vi "PDE_Cal 3D Pic Color.vi"(11 "U(x, y)":dbl[](array[numeric])) -> (3 "Color Array":T1[](array[typedef]))   [LabVIEW 2020, in "NI_PDE.lvlib"]
uses:
  <vilib>/gmath/NI_PDE.lvlib
  <vilib>/Utility/miscctls.llb/LVRGBAColorTypeDef.ctl
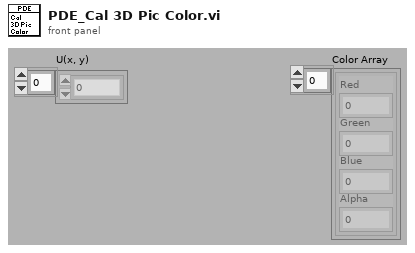
[diagram p1: front panel]
types:
  T1 = typedef "LVRGBAColorTypeDef.ctl" = cluster{"Red":sgl, "Green":sgl, "Blue":sgl, "Alpha":sgl}
  T2 = cluster{"[0]":dbl, "[1]":dbl, "[2]":dbl, "[3]":dbl}
  T3 = cluster{"[0]":dbl, "[1]":dbl, "[2]":dbl, "[3]":dbl}[]
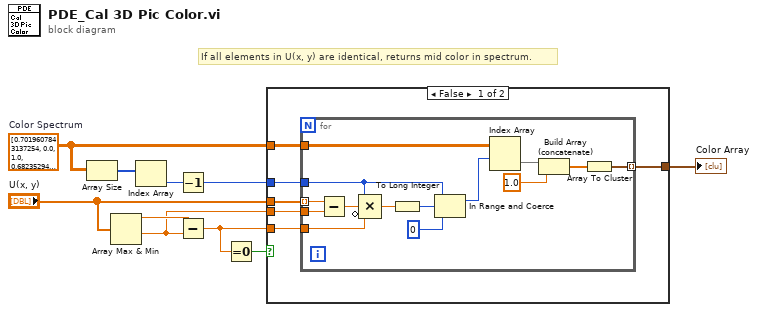
[diagram p0: block diagram]
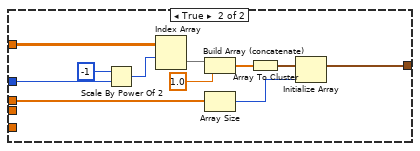
[diagram p2: hidden frame]
diagram:
  w1 = dbl[][] [[0.7019607843137254, 0.0, 1.0], [0.6823529411764706, 0.0, 1.0], [0.6666666666666666, 0.0, 1.0], [0.6470588235294118, 0.0, 1.0], [0.6313725490196078, 0.0, 1.0], [0.611764705882353, 0.0, 1.0], [0.596078431372549, 0.0, 1.0], [0.5803921568627451, 0.0, 1.0], [0.5607843137254902, 0.0, 1.0], [0.5450980392156862, 0.0, 1.0], [0.5254901960784314, 0.0, 1.0], [0.5098039215686274, 0.0, 1.0], [0.49411764705882355, 0.0, 1.0], [0.4745098039215686, 0.0, 1.0], [0.4588235294117647, 0.0, 1.0], [0.44313725490196076, 0.0, 1.0], [0.4235294117647059, 0.0, 1.0], [0.40784313725490196, 0.0, 1.0], [0.38823529411764707, 0.0, 1.0], [0.37254901960784315, 0.0, 1.0], [0.35294117647058826, 0.0, 1.0], [0.33725490196078434, 0.0, 1.0], [0.3215686274509804, 0.0, 1.0], [0.30196078431372547, 0.0, 1.0], [0.28627450980392155, 0.0, 1.0], [0.26666666666666666, 0.0, 1.0], [0.25098039215686274, 0.0, 1.0], [0.23529411764705882, 0.0, 1.0], [0.21568627450980393, 0.0, 1.0], [0.2, 0.0, 1.0], [0.1803921568627451, 0.0, 1.0], [0.16470588235294117, 0.0, 1.0], [0.14901960784313725, 0.0, 1.0], [0.12941176470588237, 0.0, 1.0], [0.11372549019607843, 0.0, 1.0], [0.09411764705882353, 0.0, 1.0], [0.0784313725490196, 0.0, 1.0], [0.06274509803921569, 0.0, 1.0], [0.043137254901960784, 0.0, 1.0], [0.027450980392156862, 0.0, 1.0], [0.00784313725490196, 0.0, 1.0], [0.0, 0.00784313725490196, 1.0], [0.0, 0.023529411764705882, 1.0], [0.0, 0.043137254901960784, 1.0], [0.0, 0.058823529411764705, 1.0], [0.0, 0.0784313725490196, 1.0], [0.0, 0.09411764705882353, 1.0], [0.0, 0.10980392156862745, 1.0], [0.0, 0.12941176470588237, 1.0], [0.0, 0.1450980392156863, 1.0], [0.0, 0.16470588235294117, 1.0], [0.0, 0.1803921568627451, 1.0], [0.0, 0.19607843137254902, 1.0], [0.0, 0.21568627450980393, 1.0], [0.0, 0.23137254901960785, 1.0], [0.0, 0.25098039215686274, 1.0], [0.0, 0.26666666666666666, 1.0], [0.0, 0.2823529411764706, 1.0], [0.0, 0.30196078431372547, 1.0], [0.0, 0.3176470588235294, 1.0], [0.0, 0.33725490196078434, 1.0], [0.0, 0.35294117647058826, 1.0], [0.0, 0.3686274509803922, 1.0], [0.0, 0.38823529411764707, 1.0], [0.0, 0.403921568627451, 1.0], [0.0, 0.4235294117647059, 1.0], [0.0, 0.4392156862745098, 1.0], [0.0, 0.4549019607843137, 1.0], [0.0, 0.4745098039215686, 1.0], [0.0, 0.49019607843137253, 1.0], [0.0, 0.5098039215686274, 1.0], [0.0, 0.5254901960784314, 1.0], [0.0, 0.5411764705882353, 1.0], [0.0, 0.5607843137254902, 1.0], [0.0, 0.5764705882352941, 1.0], [0.0, 0.596078431372549, 1.0], [0.0, 0.611764705882353, 1.0], [0.0, 0.6274509803921569, 1.0], [0.0, 0.6470588235294118, 1.0], [0.0, 0.6627450980392157, 1.0], [0.0, 0.6823529411764706, 1.0], [0.0, 0.6980392156862745, 1.0], [0.0, 0.7137254901960784, 1.0], [0.0, 0.7333333333333333, 1.0], [0.0, 0.7490196078431373, 1.0], [0.0, 0.7686274509803922, 1.0], [0.0, 0.7843137254901961, 1.0], [0.0, 0.8, 1.0], [0.0, 0.8196078431372549, 1.0], [0.0, 0.8352941176470589, 1.0], [0.0, 0.8549019607843137, 1.0], [0.0, 0.8705882352941177, 1.0], [0.0, 0.8862745098039215, 1.0], [0.0, 0.9058823529411765, 1.0], [0.0, 0.9215686274509803, 1.0], [0.0, 0.9411764705882353, 1.0], [0.0, 0.9568627450980393, 1.0], [0.0, 0.9725490196078431, 1.0], [0.0, 0.9921568627450981, 1.0], [0.0, 1.0, 0.9921568627450981], [0.0, 1.0, 0.9725490196078431], [0.0, 1.0, 0.9568627450980393], [0.0, 1.0, 0.9411764705882353], [0.0, 1.0, 0.9215686274509803], [0.0, 1.0, 0.9058823529411765], [0.0, 1.0, 0.8862745098039215], [0.0, 1.0, 0.8705882352941177], [0.0, 1.0, 0.8549019607843137], [0.0, 1.0, 0.8352941176470589], [0.0, 1.0, 0.8196078431372549], [0.0, 1.0, 0.8], [0.0, 1.0, 0.7843137254901961], [0.0, 1.0, 0.7686274509803922], [0.0, 1.0, 0.7490196078431373], [0.0, 1.0, 0.7333333333333333], [0.0, 1.0, 0.7137254901960784], [0.0, 1.0, 0.6980392156862745], [0.0, 1.0, 0.6823529411764706], [0.0, 1.0, 0.6627450980392157], [0.0, 1.0, 0.6470588235294118], [0.0, 1.0, 0.6274509803921569], [0.0, 1.0, 0.611764705882353], [0.0, 1.0, 0.596078431372549], [0.0, 1.0, 0.5764705882352941], [0.0, 1.0, 0.5607843137254902], [0.0, 1.0, 0.5411764705882353], [0.0, 1.0, 0.5254901960784314], [0.0, 1.0, 0.5098039215686274], [0.0, 1.0, 0.49019607843137253], [0.0, 1.0, 0.4745098039215686], [0.0, 1.0, 0.4549019607843137], [0.0, 1.0, 0.4392156862745098], [0.0, 1.0, 0.4235294117647059], [0.0, 1.0, 0.403921568627451], [0.0, 1.0, 0.38823529411764707], [0.0, 1.0, 0.3686274509803922], [0.0, 1.0, 0.35294117647058826], [0.0, 1.0, 0.33725490196078434], [0.0, 1.0, 0.3176470588235294], [0.0, 1.0, 0.30196078431372547], [0.0, 1.0, 0.2823529411764706], [0.0, 1.0, 0.26666666666666666], [0.0, 1.0, 0.25098039215686274], [0.0, 1.0, 0.23137254901960785], [0.0, 1.0, 0.21568627450980393], [0.0, 1.0, 0.19607843137254902], [0.0, 1.0, 0.1803921568627451], [0.0, 1.0, 0.16470588235294117], [0.0, 1.0, 0.1450980392156863], [0.0, 1.0, 0.12941176470588237], [0.0, 1.0, 0.11372549019607843], [0.0, 1.0, 0.09411764705882353], [0.0, 1.0, 0.0784313725490196], [0.0, 1.0, 0.058823529411764705], [0.0, 1.0, 0.043137254901960784], [0.0, 1.0, 0.023529411764705882], [0.0, 1.0, 0.00784313725490196], [0.00784313725490196, 1.0, 0.0], [0.027450980392156862, 1.0, 0.0], [0.043137254901960784, 1.0, 0.0], [0.06274509803921569, 1.0, 0.0], [0.0784313725490196, 1.0, 0.0], [0.09411764705882353, 1.0, 0.0], [0.11372549019607843, 1.0, 0.0], [0.12941176470588237, 1.0, 0.0], [0.14901960784313725, 1.0, 0.0], [0.16470588235294117, 1.0, 0.0], [0.1803921568627451, 1.0, 0.0], [0.2, 1.0, 0.0], [0.21568627450980393, 1.0, 0.0], [0.23529411764705882, 1.0, 0.0], [0.25098039215686274, 1.0, 0.0], [0.26666666666666666, 1.0, 0.0], [0.28627450980392155, 1.0, 0.0], [0.30196078431372547, 1.0, 0.0], [0.3215686274509804, 1.0, 0.0], [0.33725490196078434, 1.0, 0.0], [0.35294117647058826, 1.0, 0.0], [0.37254901960784315, 1.0, 0.0], [0.38823529411764707, 1.0, 0.0], [0.40784313725490196, 1.0, 0.0], [0.4235294117647059, 1.0, 0.0], [0.4392156862745098, 1.0, 0.0], [0.4588235294117647, 1.0, 0.0], [0.4745098039215686, 1.0, 0.0], [0.49411764705882355, 1.0, 0.0], [0.5098039215686274, 1.0, 0.0], [0.5254901960784314, 1.0, 0.0], [0.5450980392156862, 1.0, 0.0], [0.5607843137254902, 1.0, 0.0], [0.5803921568627451, 1.0, 0.0], [0.596078431372549, 1.0, 0.0], [0.611764705882353, 1.0, 0.0], [0.6313725490196078, 1.0, 0.0], [0.6470588235294118, 1.0, 0.0], [0.6666666666666666, 1.0, 0.0], [0.6823529411764706, 1.0, 0.0], [0.6980392156862745, 1.0, 0.0], [0.7176470588235294, 1.0, 0.0], [0.7333333333333333, 1.0, 0.0], [0.7529411764705882, 1.0, 0.0], [0.7686274509803922, 1.0, 0.0], [0.7843137254901961, 1.0, 0.0], [0.803921568627451, 1.0, 0.0], [0.8196078431372549, 1.0, 0.0], [0.8392156862745098, 1.0, 0.0], [0.8549019607843137, 1.0, 0.0], [0.8705882352941177, 1.0, 0.0], [0.8901960784313725, 1.0, 0.0], [0.9058823529411765, 1.0, 0.0], [0.9254901960784314, 1.0, 0.0], [0.9411764705882353, 1.0, 0.0], [0.9568627450980393, 1.0, 0.0], [0.9764705882352941, 1.0, 0.0], [0.9921568627450981, 1.0, 0.0], [1.0, 0.9882352941176471, 0.0], [1.0, 0.9725490196078431, 0.0], [1.0, 0.9568627450980393, 0.0], [1.0, 0.9372549019607843, 0.0], [1.0, 0.9215686274509803, 0.0], [1.0, 0.9019607843137255, 0.0], [1.0, 0.8862745098039215, 0.0], [1.0, 0.8705882352941177, 0.0], [1.0, 0.8509803921568627, 0.0], [1.0, 0.8352941176470589, 0.0], [1.0, 0.8156862745098039, 0.0], [1.0, 0.8, 0.0], [1.0, 0.7843137254901961, 0.0], [1.0, 0.7647058823529411, 0.0], [1.0, 0.7490196078431373, 0.0], [1.0, 0.7294117647058823, 0.0], [1.0, 0.7137254901960784, 0.0], [1.0, 0.6980392156862745, 0.0], [1.0, 0.6784313725490196, 0.0], [1.0, 0.6627450980392157, 0.0], [1.0, 0.6431372549019608, 0.0], [1.0, 0.6274509803921569, 0.0], [1.0, 0.611764705882353, 0.0], [1.0, 0.592156862745098, 0.0], [1.0, 0.5764705882352941, 0.0], [1.0, 0.5568627450980392, 0.0], [1.0, 0.5411764705882353, 0.0], [1.0, 0.5254901960784314, 0.0], [1.0, 0.5058823529411764, 0.0], [1.0, 0.49019607843137253, 0.0], [1.0, 0.47058823529411764, 0.0], [1.0, 0.4549019607843137, 0.0], [1.0, 0.4392156862745098, 0.0], [1.0, 0.4196078431372549, 0.0], [1.0, 0.403921568627451, 0.0], [1.0, 0.3843137254901961, 0.0], [1.0, 0.3686274509803922, 0.0], [1.0, 0.35294117647058826, 0.0], [1.0, 0.3333333333333333, 0.0], [1.0, 0.3176470588235294, 0.0], [1.0, 0.2980392156862745, 0.0]]  # Color Spectrum
  # "If all elements in U(x, y) are identical, returns mid color in spectrum."
  n1 = Array Size(array=w1) -> (size(s)=w8:i32[])
  n2 = Array Max & Min(array="U(x, y)") -> (max value=w10:dbl, min value=w9:dbl)  [unwired: 2 out]
  n3 = Index Array(array=w8) -> (element=w7:i32)  [unwired: 1 in]
  n4 = Decrement(x=w7) -> (x-1=w6:i32)
  n5 = Subtract(x=w10, y=w9) -> (x-y=w5:dbl)
  n6 = Equal To 0?(x=w5) -> (x = 0?=w4:bool)
  n7 = case shown="False" w4 {
    tunnel: w9 -> [w16 _]
    tunnel: w5 -> [w15 _]
    tunnel: w1 -> [w14 w36]
    tunnel: w6 -> [w13 w40]
    tunnel: [w12 w31] -> w3
    tunnel: "U(x, y)" -> [w11 w34]
    frame False {
      n8 = for {
        tunnel: w11 -> [w30] mode=indexing
        tunnel: w16 -> [w29]
        tunnel: w15 -> [w27]
        tunnel: [w22] -> w12 mode=indexing
        tunnel: w14 -> [w26]
        tunnel: w13 -> [w19]
        n9 = Subtract(x=w30, y=w29) -> (x-y=w28:dbl)
        n10 = Compound Arithmetic op=MULTIPLY(w19, w28, invert w27) -> (w21:dbl)
        n11 = To Long Integer(number=w21) -> (32bit integer=w17:i32)
        n12 = In Range and Coerce(upper limit=w19, x=w17, lower limit=0) -> (coerced(x)=w18:i32)  [unwired: 1 out]
        n13 = Index Array(array=w26, index (row)=w18) -> (element=w25:dbl[])  [unwired: 1 in]
        n14 = Build Array (concatenate)(w25, 1.0) -> (w23:dbl[])
        n15 = Array To Cluster(array=w23) -> (cluster=w22:T2)
      }
    }
    frame True {
      n16 = Scale By Power Of 2(n=-1, x=w40) -> (x*2^n=w35:i32)
      n17 = Index Array(array=w36, index (row)=w35) -> (element=w39:dbl[])  [unwired: 1 in]
      n18 = Build Array (concatenate)(w39, 1.0) -> (w37:dbl[])
      n19 = Array Size(array=w34) -> (size(s)=w32:i32)
      n20 = Array To Cluster(array=w37) -> (cluster=w33:T2)
      n21 = Initialize Array(w33, w32) -> (w31:T3)
    }
  }
  "Color Array" <- w3
